vi "Cypher XY LVDT Parameters.vi"() -> ()   [LabVIEW 2013]
panel:
  in  "Cypher YLVDT Offset":dbl=-0.51
  in  "Cypher XLVDT Offset":dbl=-0.34
  in  "Cypher YLVDT Sens":dbl=7.2348e-06
  in  "Cypher XLVDT Sens":dbl=7.5725e-06
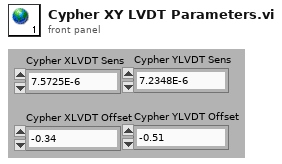
[diagram p1: front panel]
diagram:
